vi "mean_plot.vi"(7 "ref_picture":refnum<vi>, 8 "error in":errorcluster, 10 "channels":cluster{"samples":T1[]}[](array[cluster]), 11 "plot_properties":T2={"x_axis"={"min"=nan, "max"=nan, "label"="", "scale"=enum."Default"}, "y_axis"={"min"=nan, "max"=nan, "label"="", "scale"=enum."Default"}, "y multiplier"=0.0, "alpha"=0.0, "base_tag"="", "itens_base_name"="", "graph_title"="", "plot_names"=[], "plot_all"=FALSE}) -> (0 "error out":errorcluster, 2 "mean_curves":cluster{"freqs":dbl[], "Array":dbl[]}[](array[cluster]), 3 "graph":picture)   [LabVIEW 2016]
uses:
  plot_props.ctl
  axis_props.ctl
  <vilib>/Heliosphere Research LLC/Advanced Plotting Toolkit/api_core/NewPlotScales.ctl
  data_mean_plot.ctl
  <vilib>/Heliosphere Research LLC/Advanced Plotting Toolkit/Advanced Plotting Toolkit.lvlib
panel:
  out "plot_transparent":cluster{"freqs":dbl[], dbl[]}[](graph)
  out "plot":cluster{"freqs":dbl[], dbl[]}[](graph) caption="Inertância média"
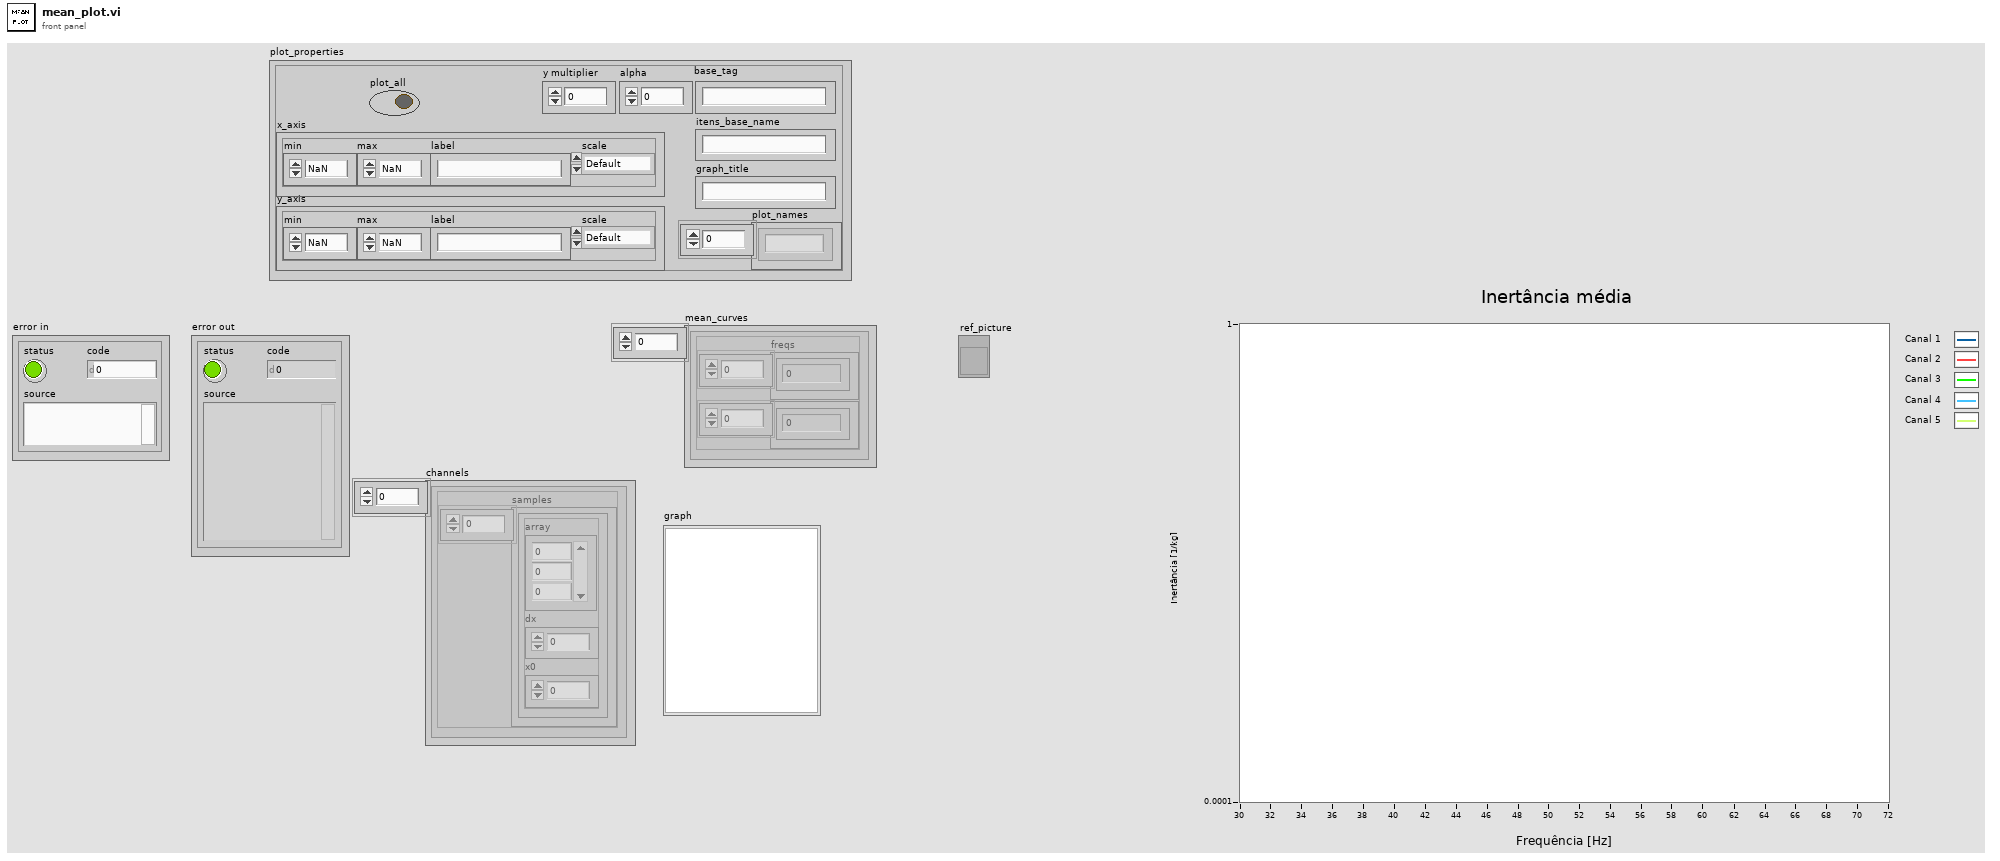
[diagram p1: front panel]
types:
  T1 = typedef "data_mean_plot.ctl" = cluster{"array":dbl[], "dx":dbl, "x0":dbl}
  T2 = typedef "plot_props.ctl" = cluster{"x_axis":T3, "y_axis":T3, "y multiplier":dbl, "alpha":dbl, "base_tag":string, "itens_base_name":string, "graph_title":string, "plot_names":string[], "plot_all":bool}
  T3 = typedef "axis_props.ctl" = cluster{"min":dbl, "max":dbl, "label":string, "scale":T4}
  T4 = typedef "Advanced Plotting Toolkit.lvlib/NewPlotScales.ctl" = enum16{"Default", "Linear", "Log", "Symlog"}
  T5 = typedef "LVBoundsTypeDef.ctl" = cluster{"Width":u32, "Height":u32}
  T6 = typedef "imagedata.ctl" = cluster{"image type":i32, "image depth":i32, "image":u8[], "mask":u8[], "colors":u32[], "Rectangle":cluster{"left":i16, "top":i16, "right":i16, "bottom":i16}}
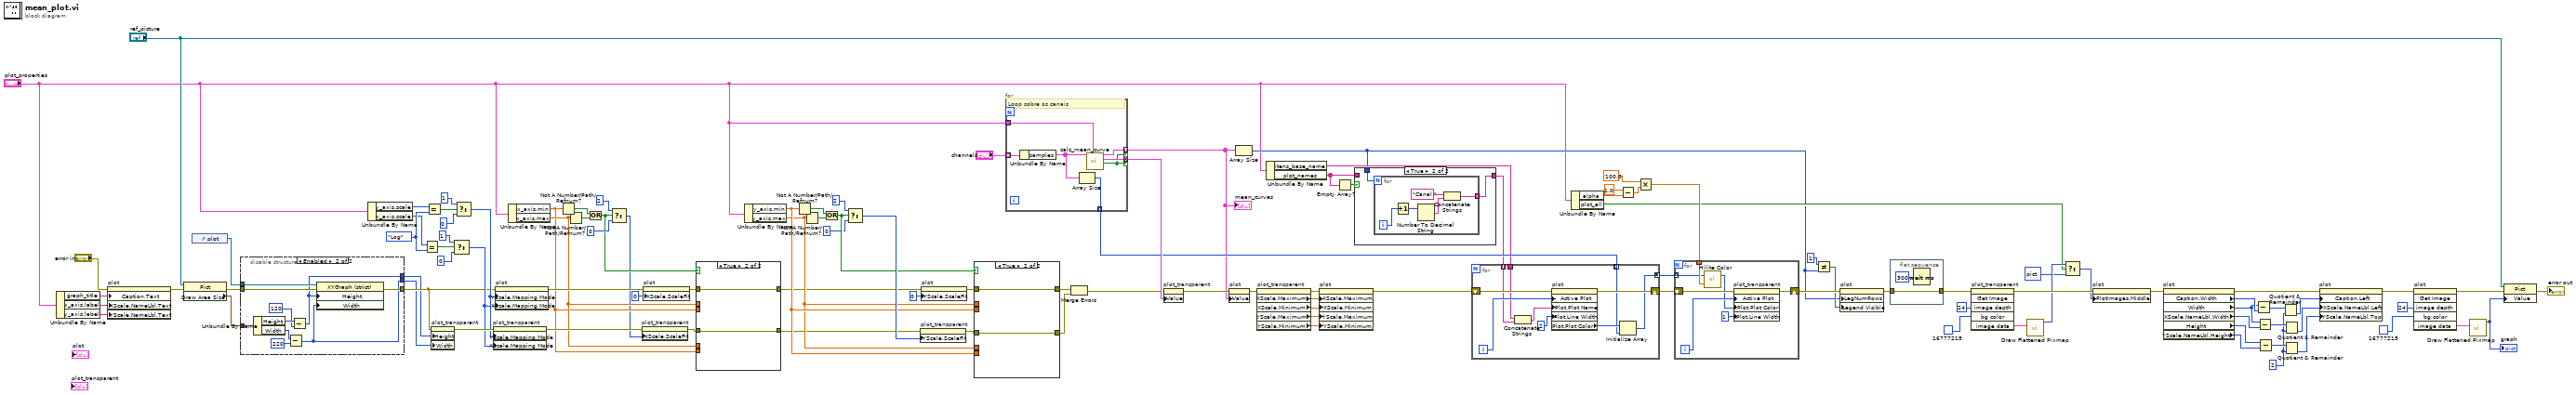
[diagram p0: block diagram]
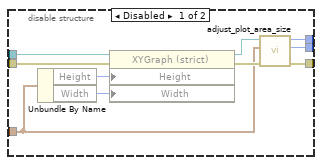
[diagram p2: hidden frame]
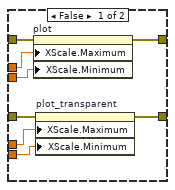
[diagram p4: hidden frame]
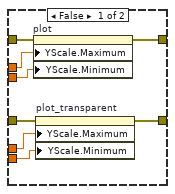
[diagram p5: hidden frame]
diagram:
  w30 = u32 2 ("y")
  w106 = NewPlotScales."Log" ("y")
  n1 = Unbundle By Name("plot_properties") -> ("graph_title"=w68:string, "x_axis.label"=w67:string, "y_axis.label"=w66:string)
  n2 = property on="plot" class="XYGraph (strict)"(error in="error in", "Caption.Text"=w68, "XScale.NameLbl.Text"=w67, "YScale.NameLbl.Text"=w66) -> (error out=w17:errorcluster)  [unwired: 1 in, 1 out]
  n3 = property class="Pict"(reference="ref_picture", error in=w17) -> (error out=w11:errorcluster, "Draw Area Size"=w10:T5)  [unwired: 1 out]
  n4 = control-ref of="plot"() -> (w12:refnum<vi>)
  n5 = disable-structure shown="Enabled" {
    disable-tunnel: [w122 w129] -> w53
    disable-tunnel: [w121 w123] -> w52
    disable-tunnel: [w120 w124] -> w51
    disable-tunnel: w12 -> [w119 w131]
    disable-tunnel: w11 -> [w117 w130]
    disable-tunnel: w10 -> [w115 w132]
    frame Disabled {
      n6 = Unbundle By Name(w115) -> ("Height"=w114:u32, "Width"=w113:u32)
      n7 = property on="Property Node" class="XYGraph (strict)"(reference=w119, error in=w117, "Height"=w114, "Width"=w113) -> (reference out=w118:refnum<vi>, error out=w116:errorcluster)
      n8 = call "adjust_plot_area_size.vi"("error in"=w116, "Draw Area Size"=w115, "ref"=w118) -> ("error out"=w122:errorcluster, "final_width"=w120:u32, "final_height"=w121:u32)  [unwired: 6 in]
    }
    frame Enabled {
      n9 = Unbundle By Name(w132) -> ("Height"=w128:u32, "Width"=w127:u32)
      n10 = Subtract(x=w127, y=u32 220) -> (x-y=w124:u32)
      n11 = Subtract(x=w128, y=u32 120) -> (x-y=w123:u32)
      n12 = property on="Property Node" class="XYGraph (strict)"(reference=w131, error in=w130, "Height"=w123, "Width"=w124) -> (error out=w129:errorcluster)  [unwired: 1 out]
    }
  }
  n13 = Unbundle By Name("plot_properties") -> ("y_axis.scale"=w112:T4, "x_axis.scale"=w105:T4)
  n14 = Equal?(x=w105, y=w106) -> (x = y?=w107:bool)
  n15 = Equal?(x=w112, y=w106) -> (x = y?=w111:bool)
  n16 = property on="plot_transparent" class="XYGraph (strict)"(error in=w53, "Height"=w52, "Width"=w51) -> (error out=w103:errorcluster)  [unwired: 1 in, 1 out]
  n17 = Select(t=u8 1 ("Y Scale.Mapping Mode"), s=w107, f=u8 0 ("Y Scale.Mapping Mode")) -> (s? t:f=w101:u8)
  n18 = Select(t=u8 1 ("Y Scale.Mapping Mode"), s=w111, f=u8 0 ("Y Scale.Mapping Mode")) -> (s? t:f=w102:u8)
  n19 = property on="plot_transparent" class="XYGraph (strict)"(error in=w103, "YScale.Mapping Mode"=w102, "XScale.Mapping Mode"=w101) -> (error out=w92:errorcluster)  [unwired: 1 in, 1 out]
  n20 = property on="plot" class="XYGraph (strict)"(error in=w53, "YScale.Mapping Mode"=w102, "XScale.Mapping Mode"=w101) -> (error out=w96:errorcluster)  [unwired: 1 in, 1 out]
  n21 = Unbundle By Name("plot_properties") -> ("x_axis.min"=w90:dbl, "x_axis.max"=w91:dbl)
  n22 = Not A Number/Path/Refnum?(number/path/refnum=w90) -> (NaN/Path/Refnum?=w99:bool)
  n23 = Not A Number/Path/Refnum?(number/path/refnum=w91) -> (NaN/Path/Refnum?=w100:bool)
  n24 = Or(x=w99, y=w100) -> (x .or. y?=w94:bool)
  n25 = Select(t=u8 2 ("X Scale.Scale Fit"), s=w94, f=u8 0 ("X Scale.Scale Fit")) -> (s? t:f=w89:u8)
  n26 = property on="plot_transparent" class="XYGraph (strict)"(error in=w92, "XScale.ScaleFit"=w89) -> (error out=w93:errorcluster)  [unwired: 1 in, 1 out]
  n27 = property on="plot" class="XYGraph (strict)"(error in=w96, "XScale.ScaleFit"=u8 0 ("X Scale.Scale Fit")) -> (error out=w95:errorcluster)  [unwired: 1 in, 1 out]
  n28 = case shown="True" w94 {
    tunnel: w95 -> [w140 w142]
    tunnel: w91 -> [w139 _]
    tunnel: w90 -> [w138 _]
    tunnel: w93 -> [w135 w141]
    tunnel: w91 -> [w136 _]
    tunnel: w90 -> [w137 _]
    tunnel: [w134 w142] -> w78
    tunnel: [w133 w141] -> w77
    frame False {
      n29 = property on="plot" class="XYGraph (strict)"(error in=w140, "XScale.Maximum"=w139, "XScale.Minimum"=w138) -> (error out=w134:errorcluster)  [unwired: 1 in, 1 out]
      n30 = property on="plot_transparent" class="XYGraph (strict)"(error in=w135, "XScale.Maximum"=w136, "XScale.Minimum"=w137) -> (error out=w133:errorcluster)  [unwired: 1 in, 1 out]
    }
    frame True {
    }
  }
  n31 = Unbundle By Name("plot_properties") -> ("y_axis.min"=w87:dbl, "y_axis.max"=w86:dbl)
  n32 = Not A Number/Path/Refnum?(number/path/refnum=w87) -> (NaN/Path/Refnum?=w80:bool)
  n33 = Not A Number/Path/Refnum?(number/path/refnum=w86) -> (NaN/Path/Refnum?=w79:bool)
  n34 = Or(x=w80, y=w79) -> (x .or. y?=w84:bool)
  n35 = Select(t=u8 2 ("X Scale.Scale Fit"), s=w84, f=u8 0 ("X Scale.Scale Fit")) -> (s? t:f=w88:u8)
  n36 = property on="plot_transparent" class="XYGraph (strict)"(error in=w77, "YScale.ScaleFit"=w88) -> (error out=w85:errorcluster)  [unwired: 1 in, 1 out]
  n37 = property on="plot" class="XYGraph (strict)"(error in=w78, "YScale.ScaleFit"=u8 0 ("Y Scale.Scale Fit")) -> (error out=w83:errorcluster)  [unwired: 1 in, 1 out]
  n38 = case shown="True" w84 {
    tunnel: w83 -> [w150 w152]
    tunnel: w86 -> [w149 _]
    tunnel: w87 -> [w148 _]
    tunnel: w85 -> [w145 w151]
    tunnel: w86 -> [w146 _]
    tunnel: w87 -> [w147 _]
    tunnel: [w144 w152] -> w76
    tunnel: [w143 w151] -> w75
    frame False {
      n39 = property on="plot" class="XYGraph (strict)"(error in=w150, "YScale.Maximum"=w149, "YScale.Minimum"=w148) -> (error out=w144:errorcluster)  [unwired: 1 in, 1 out]
      n40 = property on="plot_transparent" class="XYGraph (strict)"(error in=w145, "YScale.Maximum"=w146, "YScale.Minimum"=w147) -> (error out=w143:errorcluster)  [unwired: 1 in, 1 out]
    }
    frame True {
    }
  }
  n41 = for {
    tunnel: "channels" -> [w155] mode=indexing
    tunnel: "plot_properties" -> [w153]
    tunnel: [w158] -> w6 mode=indexing if=w156
    tunnel: [w157] -> w55 mode=concatenating if=w156
    tunnel: [w159] -> w20 mode=indexing
    # "Loop sobre os canais"
    n42 = Unbundle By Name(w155) -> ("samples"=w154:T1[])
    n43 = Array Size(array=w154) -> (size(s)=w159:i32)
    n44 = call "calc_mean_curve.vi"("plot_properties"=w153, "data"=w154) -> ("valid"=w156:bool, "plots"=w157:cluster{"Ramp Pattern":dbl[], "Array":dbl[]}[], "mean_plot"=w158:cluster{"Ramp Pattern":dbl[], "Array":dbl[]})  [unwired: 7 in]
  }
  "mean_curves" <- w6
  n45 = Merge Errors(w76, w75) -> (w54:errorcluster)
  n46 = property on="plot_transparent" class="XYGraph (strict)"(error in=w54, "Value"=w55) -> (error out=w56:errorcluster)  [unwired: 1 in, 1 out]
  n47 = property on="plot" class="XYGraph (strict)"(error in=w56, "Value"=w6) -> (error out=w45:errorcluster)  [unwired: 1 in, 1 out]
  n48 = Array Size(array=w6) -> (size(s)=w5:i32)
  n49 = property on="plot_transparent" class="XYGraph (strict)"(error in=w45) -> (error out=w50:errorcluster, "XScale.Maximum"=w46:dbl, "XScale.Minimum"=w47:dbl, "YScale.Maximum"=w48:dbl, "YScale.Minimum"=w49:dbl)  [unwired: 1 in, 1 out]
  n50 = Unbundle By Name("plot_properties") -> ("itens_base_name"=w18:string, "plot_names"=w8:string[])
  n51 = property on="plot" class="XYGraph (strict)"(error in=w50, "XScale.Maximum"=w46, "XScale.Minimum"=w47, "YScale.Maximum"=w48, "YScale.Minimum"=w49) -> (error out=w44:errorcluster)  [unwired: 1 in, 1 out]
  n52 = Empty Array?(array=w8) -> (empty?=w9:bool)
  n53 = case shown="True" w9 {
    tunnel: w8 -> [w160 _]
    tunnel: [w160 w161] -> w7
    tunnel: w5 -> [_ w162]
    frame False {
    }
    frame True {
      n54 = for {
        N: w162 -> [_]
        tunnel: [w163] -> w161 mode=indexing
        i -> [w167]
        n55 = Increment(x=w167) -> (x+1=w166:i32)
        n56 = Number To Decimal String(number=w166) -> (decimal integer string=w165:string)  [unwired: 1 in]
        n57 = Concatenate Strings("Canal " ("string"), w165) -> (w163:string)
      }
    }
  }
  n58 = for {
    shift-right: [w176] -> w74
    shift-left: w44 -> [w177]
    tunnel: w20 -> [w171] mode=indexing
    tunnel: [w170] -> w19 mode=concatenating
    tunnel: w18 -> [w169]
    tunnel: w7 -> [w168] mode=indexing
    i -> [w175]
    n59 = Concatenate Strings(w169, w168) -> (w174:string)
    n60 = property on="plot" class="XYGraph (strict)"(error in=w177, "Active Plot"=w175, "Plot.Plot Name"=w174, "Plot.Line Width"=u8 2) -> (error out=w176:errorcluster, "Plot.Plot Color"=w172:u32)  [unwired: 1 in, 1 out]
    n61 = Initialize Array(w172, w171) -> (w170:u32[])
  }
  n62 = Unbundle By Name("plot_properties") -> ("alpha"=w64:dbl, "plot_all"=w23:bool)
  n63 = Subtract(x=1.0, y=w64) -> (x-y=w62:dbl)
  n64 = Multiply(x=100.0, y=w62) -> (x*y=w60:dbl)
  n65 = for {
    shift-right: [w183] -> w27
    shift-left: w74 -> [w184]
    tunnel: w60 -> [w179]
    tunnel: w19 -> [w178] mode=indexing
    i -> [w182]
    n66 = call <vilib>:"Hilite Color.vi"("Percentage(30)"=w179, "Color In"=w178) -> ("Hilite"=w180:u32)  [unwired: 1 out]
    n67 = property on="plot_transparent" class="XYGraph (strict)"(error in=w184, "Active Plot"=w182, "Plot.Plot Color"=w180, "Plot.Line Width"=u8 1) -> (error out=w183:errorcluster)  [unwired: 1 in, 1 out]
  }
  n68 = Not Equal?(x=1, y=w5) -> (x != y?=w21:bool)
  n69 = property on="plot" class="XYGraph (strict)"(error in=w27, "LegNumRows"=w5, "Legend Visible"=w21) -> (error out=w3:errorcluster)  [unwired: 1 in, 1 out]
  n70 = flat-sequence {
    tunnel: [w186] -> w4
    tunnel: w3 -> [w186]
    frame #0 {
      n71 = Wait (ms)(milliseconds to wait=u32 300) -> ()  [unwired: 1 out]
    }
  }
  n72 = invoke on="plot_transparent" class="XYGraph (strict)" method="Get Image"(error in=w4, "image depth"=24 ("Image Depth"), "bg color"=u32 16777215) -> (error out=w43:errorcluster, "image data"=w69:T6)  [unwired: 3 in, 4 out]
  n73 = call <vilib>:"Draw Flattened Pixmap.vi"("image data"=w69) -> ("new picture"=w26:picture)  [unwired: 8 in]
  n74 = Select(t=w26, s=w23, f=picture data[5B]) -> (s? t:f=w24:picture)
  n75 = property on="plot" class="XYGraph (strict)"(error in=w43, "PlotImages.Middle"=w24) -> (error out=w41:errorcluster)  [unwired: 1 in, 1 out]
  n76 = property on="plot" class="XYGraph (strict)"(error in=w41) -> (error out=w42:errorcluster, "Caption.Width"=w33:u32, "Width"=w32:u32, "XScale.NameLbl.Width"=w38:u32, "Height"=w36:u32, "YScale.NameLbl.Height"=w28:u32)  [unwired: 1 in, 1 out]
  n77 = Subtract(x=w32, y=w33) -> (x-y=w31:u32)
  n78 = Subtract(x=w32, y=w38) -> (x-y=w37:u32)
  n79 = Subtract(x=w36, y=w28) -> (x-y=w35:u32)
  n80 = Quotient & Remainder(x=w31, y=w30) -> (floor(x/y)=w29:u32)  [unwired: 1 out]
  n81 = Quotient & Remainder(x=w37, y=w30) -> (floor(x/y)=w34:u32)  [unwired: 1 out]
  n82 = Quotient & Remainder(x=w35, y=w30) -> (floor(x/y)=w39:u32)  [unwired: 1 out]
  n83 = property on="plot" class="XYGraph (strict)"(error in=w42, "Caption.Left"=w29, "XScale.NameLbl.Left"=w34, "YScale.NameLbl.Top"=w39) -> (error out=w40:errorcluster)  [unwired: 1 in, 1 out]
  n84 = invoke on="plot" class="XYGraph (strict)" method="Get Image"(error in=w40, "image depth"=24 ("Image Depth"), "bg color"=u32 16777215) -> (error out=w15:errorcluster, "image data"=w59:T6)  [unwired: 3 in, 4 out]
  n85 = call <vilib>:"Draw Flattened Pixmap.vi"("image data"=w59) -> ("new picture"=w16:picture)  [unwired: 8 in]
  "graph" <- w16
  n86 = property class="Pict"(reference="ref_picture", error in=w15, "Value"=w16) -> (error out=→"error out":errorcluster)  [unwired: 1 out]
